vi "SR_J-Check AIP buttons.vi"(8 "error in (no error)":errorcluster, 10 "RDS Msg Q in":refnum<user-event>, 11 "Joystick":T1) -> (0 "error out":errorcluster, 2 "RDS Msg Q":refnum<user-event>, 3 "Joystick Out":T1)   [LabVIEW 2015, in "Shore Library.lvlib"]
uses:
  Shore Library.lvlib
  Libraries/RDS Framework/RDS Message Class/RDS Message.lvclass
  SR-J-State.ctl
  Libraries/RDS Framework/RDS Message Class/AIP Command Control.ctl
  AIP Instrument/AIP Instrument.lvlib
  Libraries/RDS Child Messages/RDS Child Messages.lvlib
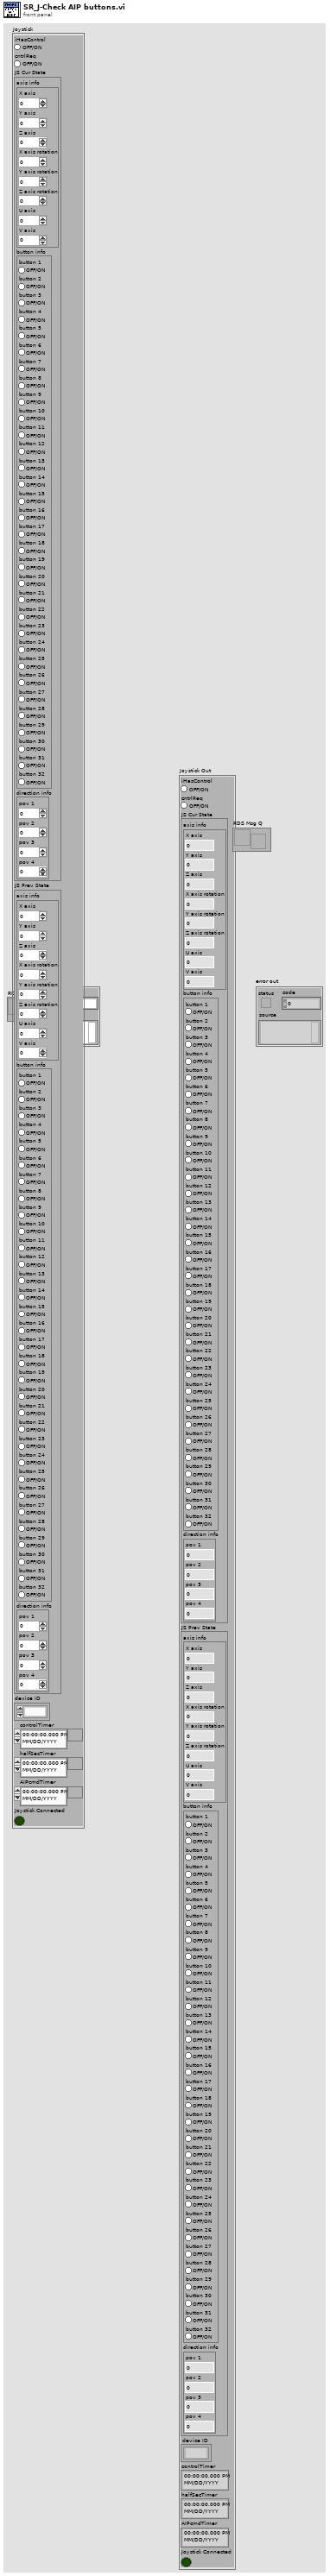
[diagram p1: front panel]
types:
  T1 = typedef "Shore Library.lvlib/SR-J-State.ctl" = cluster{"iHasControl":bool, "cntrlReq":bool, "JS Cur State":cluster{"axis info":cluster{"X axis":i32, "Y axis":i32, "Z axis":i32, "X axis rotation":i32, "Y axis rotation":i32, "Z axis rotation":i32, "U axis":i32, "V axis":i32}, "button info":cluster{"button 1":bool, "button 2":bool, "button 3":bool, "button 4":bool, "button 5":bool, "button 6":bool, "button 7":bool, "button 8":bool, "button 9":bool, "button 10":bool, "button 11":bool, "button 12":bool, "button 13":bool, "button 14":bool, "button 15":bool, "button 16":bool, "button 17":bool, "button 18":bool, "button 19":bool, "button 20":bool, "button 21":bool, "button 22":bool, "button 23":bool, "button 24":bool, "button 25":bool, "button 26":bool, "button 27":bool, "button 28":bool, "button 29":bool, "button 30":bool, "button 31":bool, "button 32":bool}, "direction info":cluster{"pov 1":i32, "pov 2":i32, "pov 3":i32, "pov 4":i32}}, "JS Prev State":cluster{"axis info":cluster{"X axis":i32, "Y axis":i32, "Z axis":i32, "X axis rotation":i32, "Y axis rotation":i32, "Z axis rotation":i32, "U axis":i32, "V axis":i32}, "button info":cluster{"button 1":bool, "button 2":bool, "button 3":bool, "button 4":bool, "button 5":bool, "button 6":bool, "button 7":bool, "button 8":bool, "button 9":bool, "button 10":bool, "button 11":bool, "button 12":bool, "button 13":bool, "button 14":bool, "button 15":bool, "button 16":bool, "button 17":bool, "button 18":bool, "button 19":bool, "button 20":bool, "button 21":bool, "button 22":bool, "button 23":bool, "button 24":bool, "button 25":bool, "button 26":bool, "button 27":bool, "button 28":bool, "button 29":bool, "button 30":bool, "button 31":bool, "button 32":bool}, "direction info":cluster{"pov 1":i32, "pov 2":i32, "pov 3":i32, "pov 4":i32}}, "device ID":refnum<k1>, "controlTimer":timestamp, "halfSecTimer":timestamp, "AIPcmdTimer":timestamp, "Joystick Connected":bool}
  T2 = typedef "RDS Child Messages.lvlib/AIP Command Control.ctl" = enum16{"Stow", "Deploy", "Stop", "Validate Sensors", "Jog Deploy FP", "Jog Stow FP", "Jog Deploy FS", "Jog Stow FS", "Jog Deploy AP", "Jog Stow AP", "Jog Deploy AS", "Jog Stow AS", "Deploy FP", "Deploy FS", "Deploy AP", "Deploy AS", "Stow FP", "Stow FS", "Stow AP", "Stow AS"}
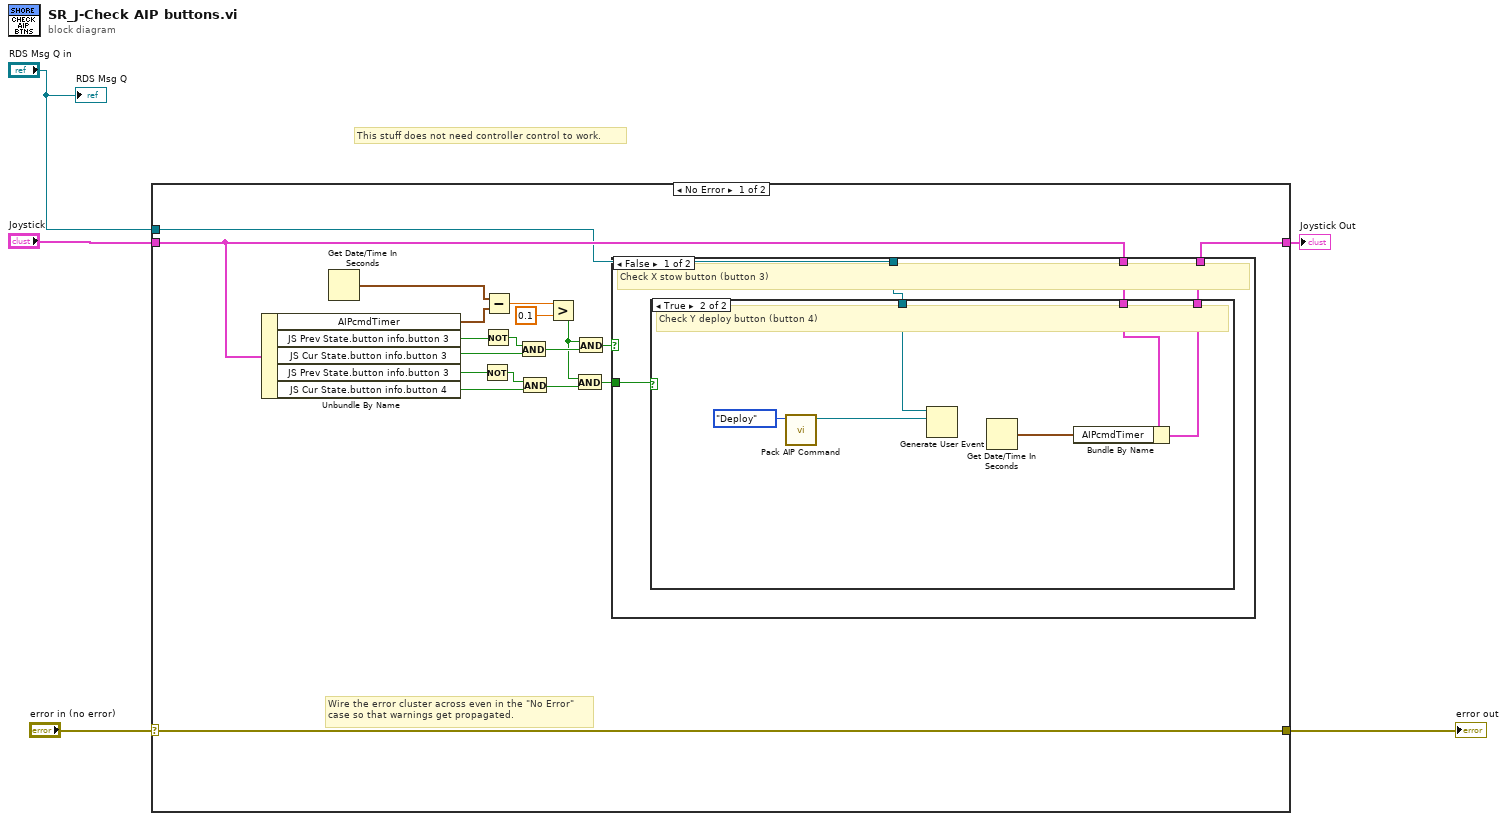
[diagram p0: block diagram]
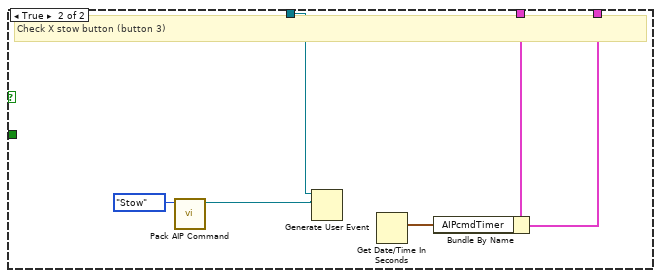
[diagram p3: hidden frame]
diagram:
  # "This stuff does not need controller control to work."
  n1 = case shown="No Error" "error in (no error)" {
    selector: "error in (no error)" -> [w24 w43]
    tunnel: [w24 w43] -> w4
    tunnel: [w7 w42] -> w1
    tunnel: "Joystick" -> [w8 w42]
    tunnel: "RDS Msg Q in" -> [w6 _]
    frame No Error {
      # "Wire the error cluster across even in the \"No Error\"\ncase so that warnings get propagated."
      n2 = Unbundle By Name(w8) -> ("AIPcmdTimer"=w18:timestamp, "JS Prev State.button info.button 3"=w23:bool, "JS Cur State.button info.button 3"=w21:bool, "JS Prev State.button info.button 3"=w14:bool, "JS Cur State.button info.button 4"=w12:bool)
      n3 = Get Date/Time In Seconds() -> (seconds since 1Jan1904=w17:timestamp)
      n4 = Not(x=w14) -> (.not. x?=w13:bool)
      n5 = Not(x=w23) -> (.not. x?=w22:bool)
      n6 = Subtract(x=w17, y=w18) -> (x-y=w16:dbl)
      n7 = And(x=w22, y=w21) -> (x .and. y?=w20:bool)
      n8 = And(x=w13, y=w12) -> (x .and. y?=w10:bool)
      n9 = Greater?(x=w16, y=0.1) -> (0:w11:bool)
      n10 = And(x=w11, y=w10) -> (x .and. y?=w9:bool)
      n11 = And(x=w11, y=w20) -> (x .and. y?=w19:bool)
      n12 = case shown="False" w19 {
        tunnel: w8 -> [w25 w38]
        tunnel: w9 -> [w28 _]
        tunnel: [w27 w40] -> w7
        tunnel: w6 -> [w26 w37]
        frame False {
          # "Check X stow button (button 3)"
          n13 = case shown="True" w28 {
            tunnel: w26 -> [_ w32]
            tunnel: [w29 w33] -> w27
            tunnel: w25 -> [w29 w31]
            frame False {
            }
            frame True {
              # "Check Y deploy button (button 4)"
              n14 = call "Pack AIP Command.vi"("AIP Command"=AIP_Command_Control."Deploy") -> ("AIP Deploy Command out"=w30:refnum<class "AIP Command.lvclass">)  [unwired: 10 in]
              n15 = Generate User Event(user event=w32, event data cluster=w30) -> ()  [unwired: 2 in, 2 out]
              n16 = Get Date/Time In Seconds() -> (seconds since 1Jan1904=w34:timestamp)
              n17 = Bundle By Name(cluster=w31, "AIPcmdTimer"=w34) -> (w33:T1)
            }
          }
        }
        frame True {
          # "Check X stow button (button 3)"
          n18 = call "Pack AIP Command.vi"("AIP Command"=AIP_Command_Control."Stow") -> ("AIP Deploy Command out"=w36:refnum<class "AIP Command.lvclass">)  [unwired: 10 in]
          n19 = Generate User Event(user event=w37, event data cluster=w36) -> ()  [unwired: 2 in, 2 out]
          n20 = Get Date/Time In Seconds() -> (seconds since 1Jan1904=w39:timestamp)
          n21 = Bundle By Name(cluster=w38, "AIPcmdTimer"=w39) -> (w40:T1)
        }
      }
    }
    frame Error {
    }
  }
  "error out" <- w4
  "Joystick Out" <- w1
  "RDS Msg Q" <- "RDS Msg Q in"
